vi "uarv7.vi"() -> ()   [LabVIEW 2023]
uses:
  perionica_states.ctl
panel:
  out "Enum":T1
  in  "Specijalno pranje":bool
  in  "Obicno pranje":bool
  out "Susenje":bool
  out "Ispiranje":bool
  out "Voskiranje":bool
  out "Samponiranje":bool
  out "Pranje sasije":bool
  in  "?":bool
  out "error out":errorcluster
  in  "error in (no error)":errorcluster
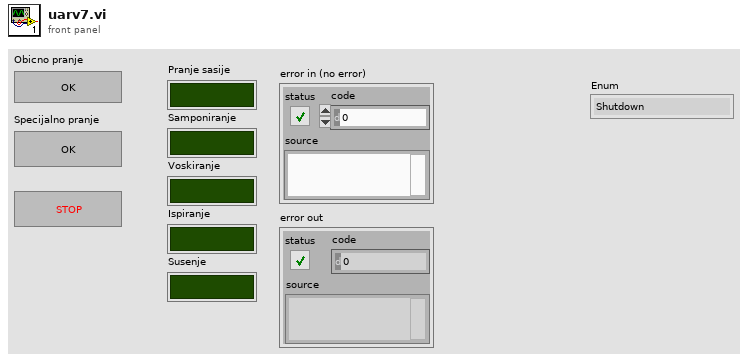
[diagram p1: front panel]
types:
  T1 = typedef "perionica_states.ctl" = enum16{"Shutdown", "Zaustavljeno", "Pranje sasije", "Samponiranje", "Voskiranje", "Ispiranje", "Susenje"}
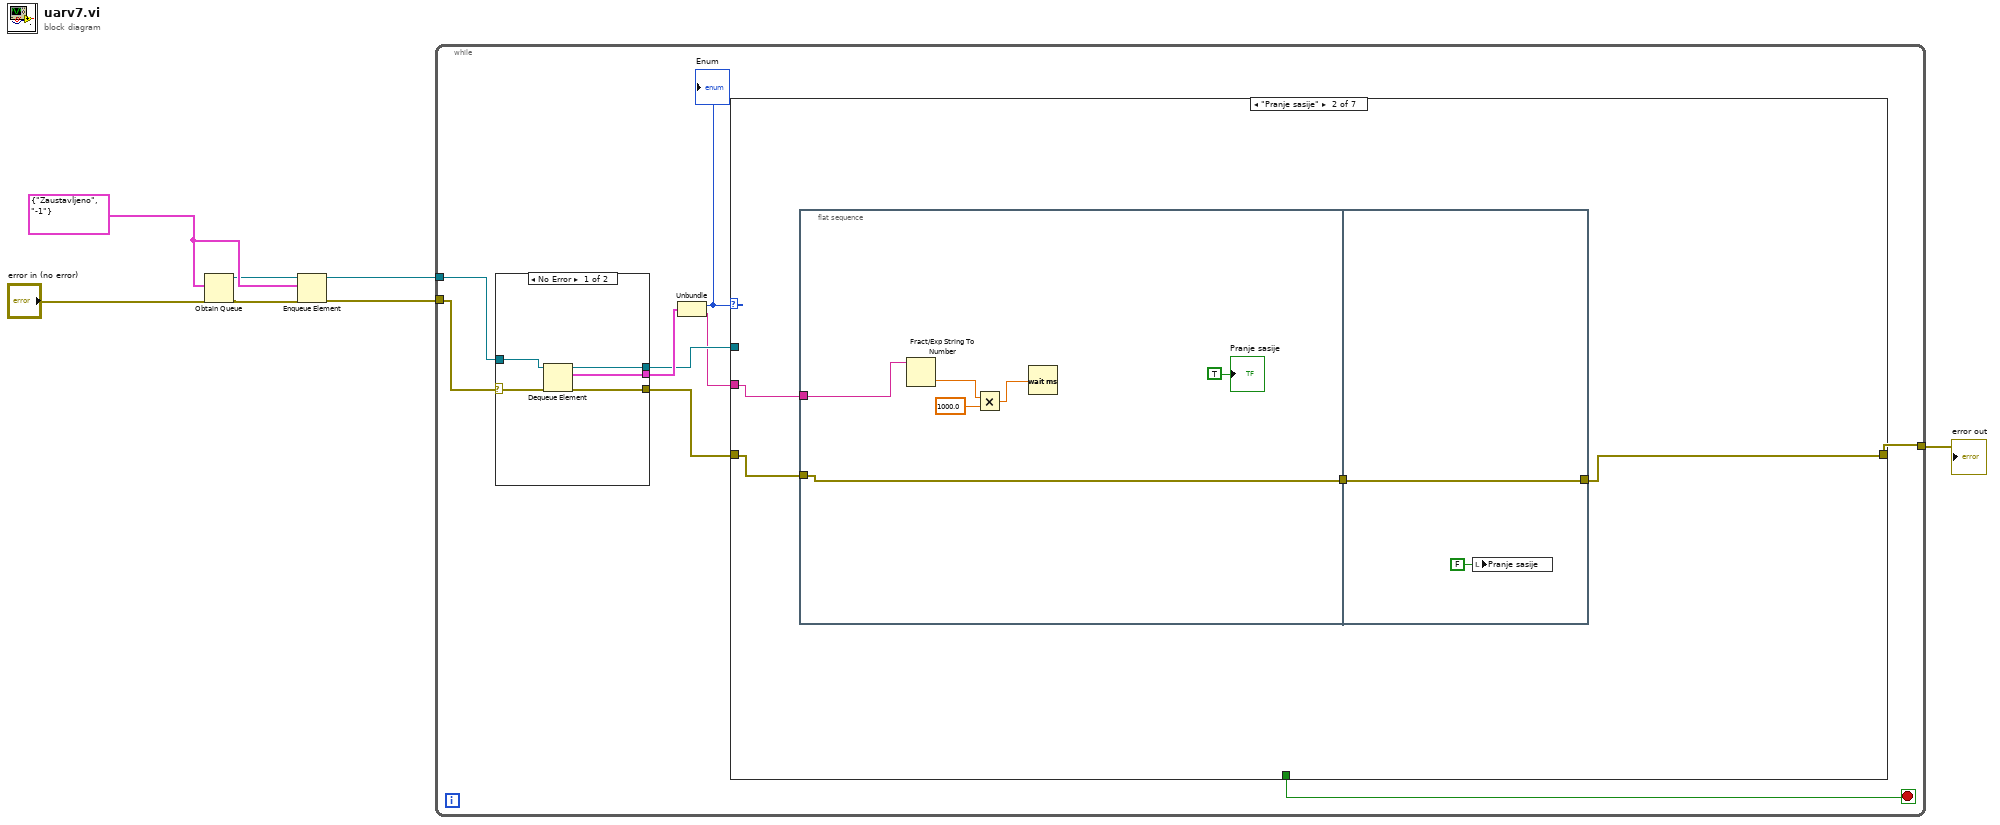
[diagram p0: block diagram]
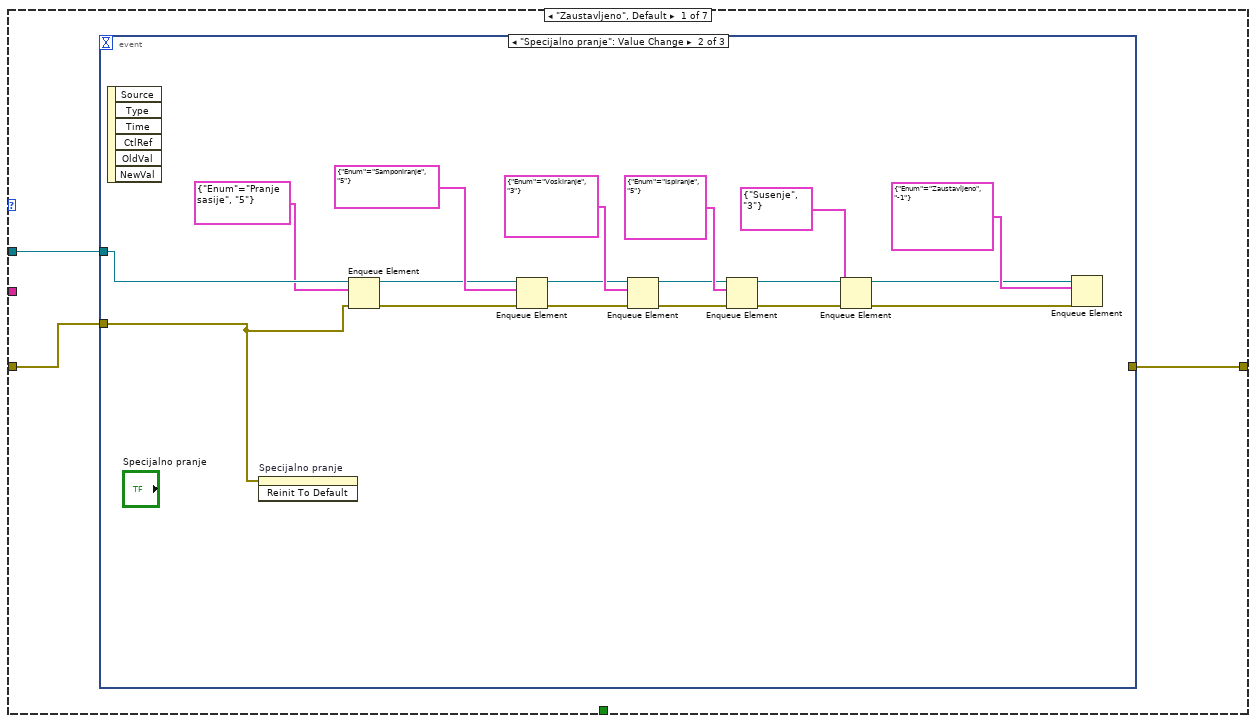
[diagram p2: hidden frame]
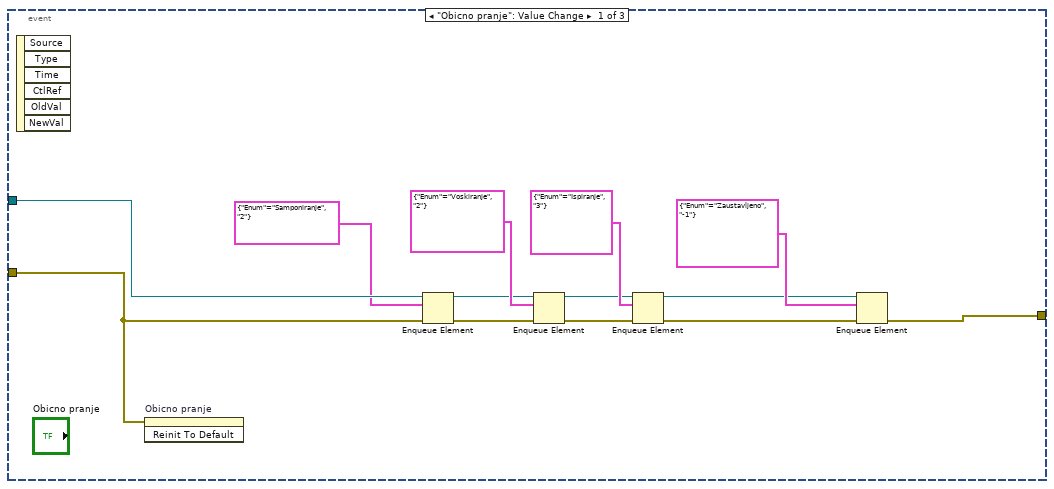
[diagram p3: hidden frame]
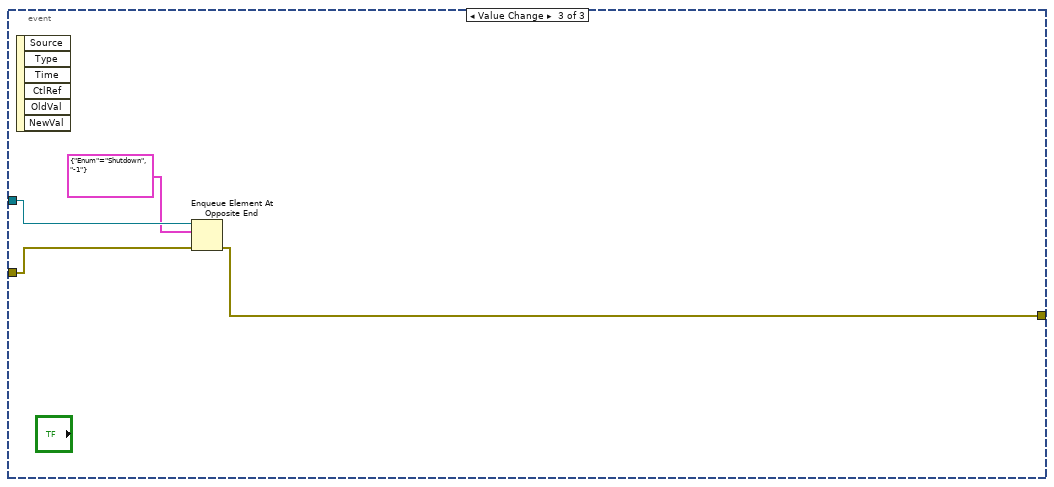
[diagram p4: hidden frame]
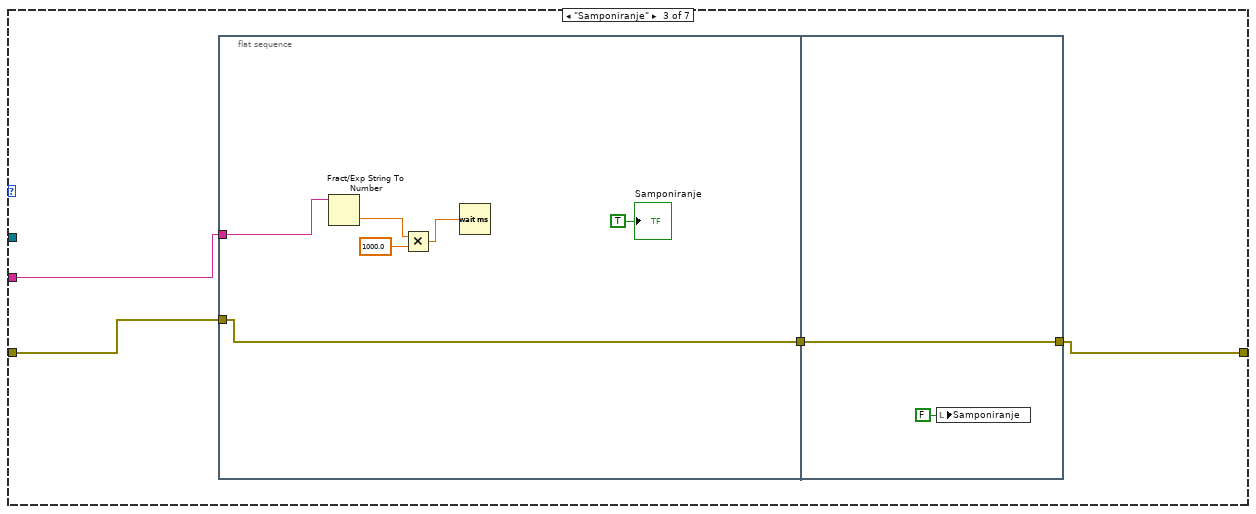
[diagram p5: hidden frame]
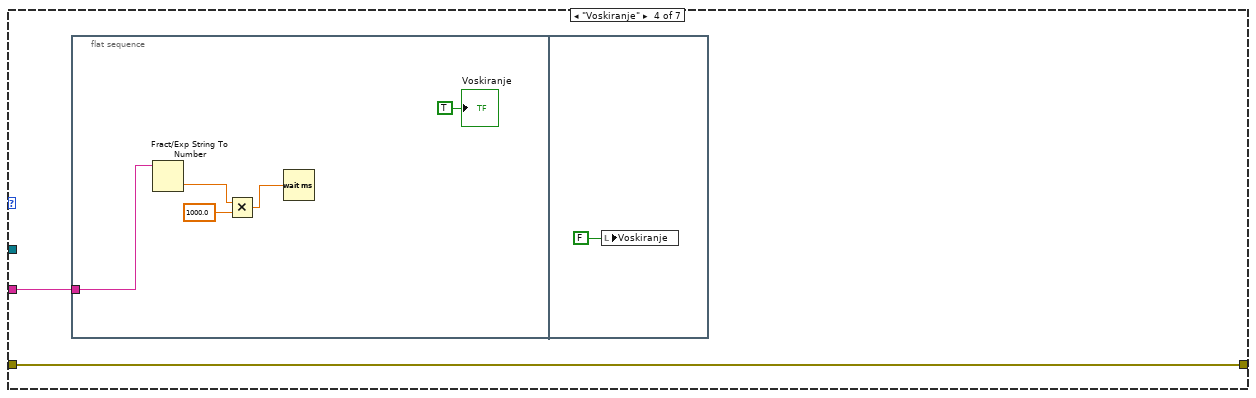
[diagram p6: hidden frame]
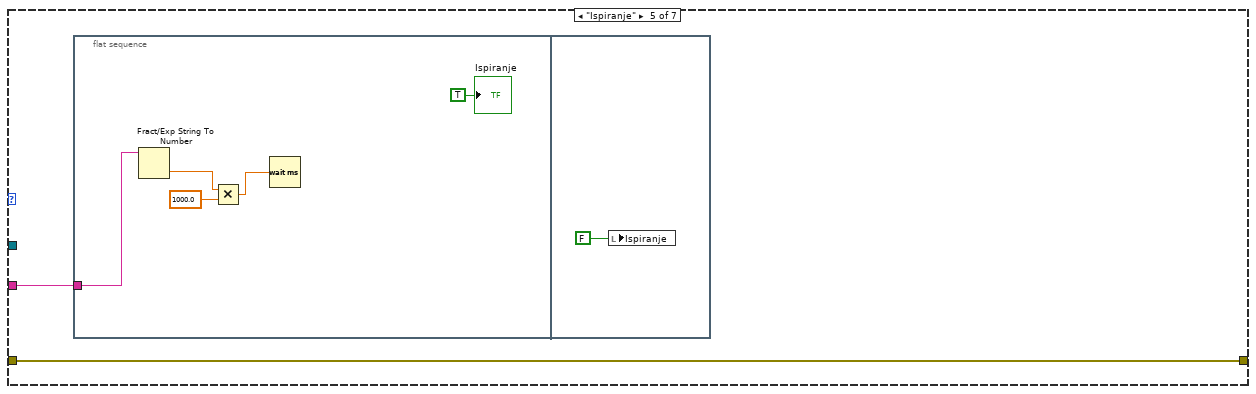
[diagram p7: hidden frame]
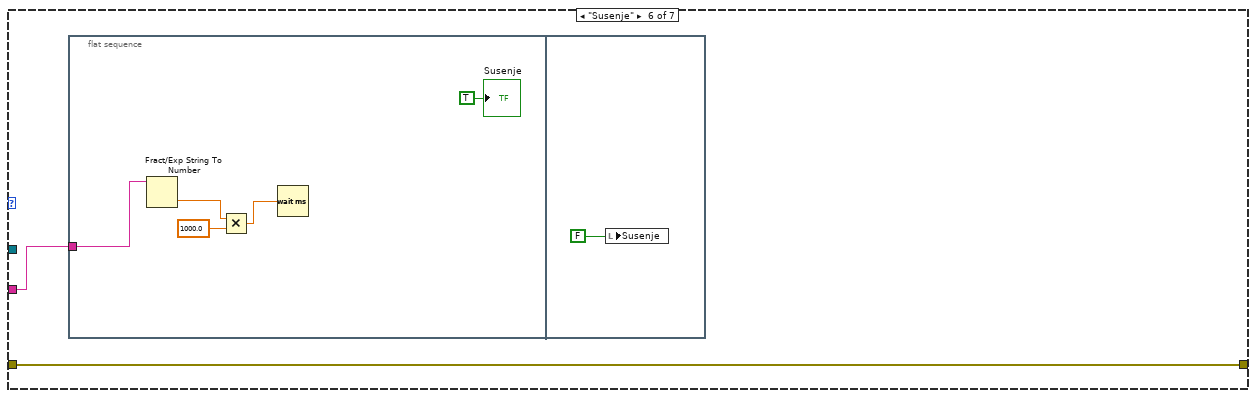
[diagram p8: hidden frame]
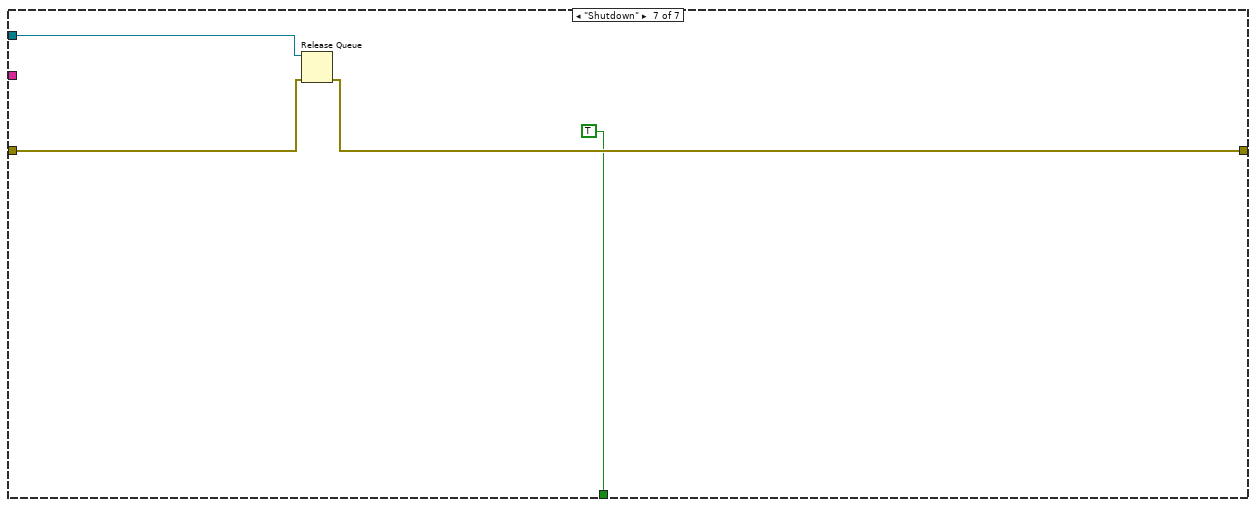
[diagram p9: hidden frame]
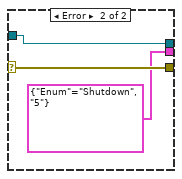
[diagram p10: hidden frame]
diagram:
  w5 = cluster{"Enum":T1, string} {"Enum"=enum."Zaustavljeno", "-1"} ("Cluster")
  n1 = Obtain Queue(element data type=w5, error in (no error)="error in (no error)") -> (queue out=w2:refnum<queue>, error out=w6:errorcluster)  [unwired: 3 in, 1 out]
  n2 = Enqueue Element(queue=w2, element=w5, error in (no error)=w6) -> (queue out=w4:refnum<queue>, error out=w3:errorcluster)  [unwired: 1 in, 1 out]
  n3 = while {
    tunnel: w4 -> [w15]
    tunnel: w3 -> [w16]
    tunnel: [w10] -> w1
    stop <- w8 stop-if-true
    n4 = case shown="No Error" w16 {
      selector: w16 -> [w110 w114]
      tunnel: w15 -> [w111 w113]
      tunnel: [w109 w113] -> w13
      tunnel: [w108 cluster{"Enum":T1, string} {"Enum"=enum."Shutdown", "5"}] -> w14
      tunnel: [w107 w114] -> w12
      frame No Error {
        n5 = Dequeue Element(queue=w111, error in (no error)=w110) -> (queue out=w109:refnum<queue>, element=w108:cluster{"Enum":T1, string}, error out=w107:errorcluster)  [unwired: 1 in, 1 out]
      }
      frame Error {
      }
    }
    n6 = Unbundle(w14) -> ("Enum"=w11:T1, w9:string)
    "Enum" <- w11
    n7 = case shown="\"Pranje sasije\"" w11 {
      tunnel: w13 -> [w19 _ _ _ _ _ w104]
      tunnel: w12 -> [w18 w57 w69 w80 w88 w96 w106]
      tunnel: [w17 w55 w67 w80 w88 w96 w105] -> w10
      tunnel: w9 -> [_ w58 w70 w79 w87 w95 _]
      tunnel: [_ _ _ _ _ _ TRUE] -> w8
      frame "Zaustavljeno", Default {
        n8 = event shown="[1] \"Specijalno pranje\": Value Change" {
          selector: _ -> [_ _ _]
          dyn-events: _ -> [_ _ _]
          timeout: _ -> [_ _ _]
          tunnel: w19 -> [w23 w40 w52]
          tunnel: w18 -> [w24 w39 w54]
          tunnel: [w31 _ w53] -> w17
          event "Obicno pranje": Value Change {
            n9 = event-data() -> ()  [unwired: 1 in, 6 out]
            n10 = invoke on="Obicno pranje" class="Bool" method="Reinit To Default"(error in=w24) -> ()  [unwired: 2 in, 3 out]
            n11 = Enqueue Element(queue=w23, element=cluster{"Enum":T1, string} {"Enum"=enum."Samponiranje", "2"}, error in (no error)=w24) -> (queue out=w26:refnum<queue>, error out=w25:errorcluster)  [unwired: 1 in, 1 out]
            n12 = Enqueue Element(queue=w26, element=cluster{"Enum":T1, string} {"Enum"=enum."Voskiranje", "2"}, error in (no error)=w25) -> (queue out=w29:refnum<queue>, error out=w28:errorcluster)  [unwired: 1 in, 1 out]
            n13 = Enqueue Element(queue=w29, element=cluster{"Enum":T1, string} {"Enum"=enum."Ispiranje", "3"}, error in (no error)=w28) -> (queue out=w21:refnum<queue>, error out=w22:errorcluster)  [unwired: 1 in, 1 out]
            n14 = Enqueue Element(queue=w21, element=cluster{"Enum":T1, string} {"Enum"=enum."Zaustavljeno", "-1"}, error in (no error)=w22) -> (error out=w31:errorcluster)  [unwired: 1 in, 2 out]
          }
          event "Specijalno pranje": Value Change {
            n15 = event-data() -> ()  [unwired: 1 in, 6 out]
            n16 = invoke on="Specijalno pranje" class="Bool" method="Reinit To Default"(error in=w39) -> ()  [unwired: 2 in, 3 out]
            n17 = Enqueue Element(queue=w40, element=cluster{"Enum":T1, string} {"Enum"=enum."Pranje sasije", "5"}, error in (no error)=w39) -> (queue out=w42:refnum<queue>, error out=w41:errorcluster)  [unwired: 1 in, 1 out]
            n18 = Enqueue Element(queue=w42, element=cluster{"Enum":T1, string} {"Enum"=enum."Samponiranje", "5"}, error in (no error)=w41) -> (queue out=w45:refnum<queue>, error out=w44:errorcluster)  [unwired: 1 in, 1 out]
            n19 = Enqueue Element(queue=w45, element=cluster{"Enum":T1, string} {"Enum"=enum."Voskiranje", "3"}, error in (no error)=w44) -> (queue out=w48:refnum<queue>, error out=w47:errorcluster)  [unwired: 1 in, 1 out]
            n20 = Enqueue Element(queue=w48, element=cluster{"Enum":T1, string} {"Enum"=enum."Ispiranje", "5"}, error in (no error)=w47) -> (queue out=w36:refnum<queue>, error out=w37:errorcluster)  [unwired: 1 in, 1 out]
            n21 = Enqueue Element(queue=w36, element=cluster{"Enum":T1, string} {"Enum"=enum."Susenje", "3"}, error in (no error)=w37) -> (queue out=w33:refnum<queue>, error out=w34:errorcluster)  [unwired: 1 in, 1 out]
            n22 = Enqueue Element(queue=w33, element=cluster{"Enum":T1, string} {"Enum"=enum."Zaustavljeno", "-1"}, error in (no error)=w34) -> ()  [unwired: 1 in, 3 out]
          }
          event Value Change {
            n23 = event-data() -> ()  [unwired: 1 in, 6 out]
            n24 = Enqueue Element At Opposite End(queue=w52, element=cluster{"Enum":T1, string} {"Enum"=enum."Shutdown", "-1"} ("Cluster"), error in (no error)=w54) -> (error out=w53:errorcluster)  [unwired: 1 in, 2 out]
          }
        }
      }
      frame "Pranje sasije" {
        n25 = flat-sequence {
          tunnel: w58 -> [w60]
          tunnel: w57 -> [w61]
          tunnel: [w61] -> w56
          tunnel: w56 -> [w65]
          tunnel: [w65] -> w55
          frame #0 {
            n26 = Fract/Exp String To Number(string=w60) -> (number=w64:dbl)  [unwired: 3 in, 1 out]
            n27 = Multiply(x=w64, y=1000.0) -> (x*y=w63:dbl)
            n28 = Wait (ms)(milliseconds to wait=w63) -> ()  [unwired: 1 out]
            "Pranje sasije" <- TRUE ("Pranje sasije")
          }
          frame #1 {
            n29 = local write "Pranje sasije"(FALSE ("Pranje sasije")) -> ()
          }
        }
      }
      frame "Samponiranje" {
        n30 = flat-sequence {
          tunnel: w70 -> [w71]
          tunnel: w69 -> [w76]
          tunnel: [w76] -> w68
          tunnel: w68 -> [w77]
          tunnel: [w77] -> w67
          frame #0 {
            n31 = Fract/Exp String To Number(string=w71) -> (number=w75:dbl)  [unwired: 3 in, 1 out]
            n32 = Multiply(x=w75, y=1000.0) -> (x*y=w74:dbl)
            n33 = Wait (ms)(milliseconds to wait=w74) -> ()  [unwired: 1 out]
            "Samponiranje" <- TRUE ("Samponiranje")
          }
          frame #1 {
            n34 = local write "Samponiranje"(FALSE ("Pranje sasije")) -> ()
          }
        }
      }
      frame "Voskiranje" {
        n35 = flat-sequence {
          tunnel: w79 -> [w81]
          frame #0 {
            n36 = Fract/Exp String To Number(string=w81) -> (number=w84:dbl)  [unwired: 3 in, 1 out]
            n37 = Multiply(x=w84, y=1000.0) -> (x*y=w83:dbl)
            n38 = Wait (ms)(milliseconds to wait=w83) -> ()  [unwired: 1 out]
            "Voskiranje" <- TRUE ("Voskiranje")
          }
          frame #1 {
            n39 = local write "Voskiranje"(FALSE ("Pranje sasije")) -> ()
          }
        }
      }
      frame "Ispiranje" {
        n40 = flat-sequence {
          tunnel: w87 -> [w89]
          frame #0 {
            n41 = Fract/Exp String To Number(string=w89) -> (number=w92:dbl)  [unwired: 3 in, 1 out]
            n42 = Multiply(x=w92, y=1000.0) -> (x*y=w91:dbl)
            n43 = Wait (ms)(milliseconds to wait=w91) -> ()  [unwired: 1 out]
            "Ispiranje" <- TRUE ("Ispiranje")
          }
          frame #1 {
            n44 = local write "Ispiranje"(FALSE ("Pranje sasije")) -> ()
          }
        }
      }
      frame "Susenje" {
        n45 = flat-sequence {
          tunnel: w95 -> [w97]
          frame #0 {
            n46 = Fract/Exp String To Number(string=w97) -> (number=w100:dbl)  [unwired: 3 in, 1 out]
            n47 = Multiply(x=w100, y=1000.0) -> (x*y=w99:dbl)
            n48 = Wait (ms)(milliseconds to wait=w99) -> ()  [unwired: 1 out]
            "Susenje" <- TRUE ("Susenje")
          }
          frame #1 {
            n49 = local write "Susenje"(FALSE ("Pranje sasije")) -> ()
          }
        }
      }
      frame "Shutdown" {
        n50 = Release Queue(queue=w104, error in (no error)=w106) -> (error out=w105:errorcluster)  [unwired: 1 in, 2 out]
      }
    }
  }
  "error out" <- w1
